vi "Halt AFM.vi"() -> ()   [LabVIEW 2017]
panel:
  in  "stop":bool
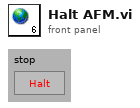
[diagram p1: front panel]
diagram:
